vi "building_timbre.vi"() -> ()   [LabVIEW 2023]
uses:
  <vilib>/Analysis/3filter.llb/Filter Passband Type.ctl
  <vilib>/express/express analysis/Spectral/Block/exnSpectralBlock spectral measurements RMS poly.vi
  <vilib>/express/express analysis/Spectral/Block/exnSpectralBlock spectral measurements RMS WFM.vi
  <vilib>/express/express analysis/Spectral/XNode/ExpressSpectralMeasurementsBlockNode.xnode
  <vilib>/Analysis/NI_AALBase.lvlib
panel:
  out "Frequency Graph":cluster{"f0":dbl, "df":dbl, "magnitude":dbl[]}[](graph)
  in  "Duration (s)":dbl=1.0
  in  "Record Sound":bool
  in  "Open File":bool
  in  "path":path
  in  "Play Recorded Sound":bool
  in  "Play Sound":bool
  in  "stop":bool
  in  "Generated Signals":T1(array[cluster]) {"Signal" items=["Sine", "Square", "Triangle", "Sawtooth"]}
  in  "?":T3={"filter type"=enum."Lowpass", "low cutoff freq"=0.12500000000000006, "high cutoff freq"=0.45000000000000007} {"high cutoff freq" format="%0.2f"; "low cutoff freq" format="%0.4f"}
  in  "Filter OFF          Filter ON":bool
  out "Waveform Graph":waveform(dbl)[](graph)
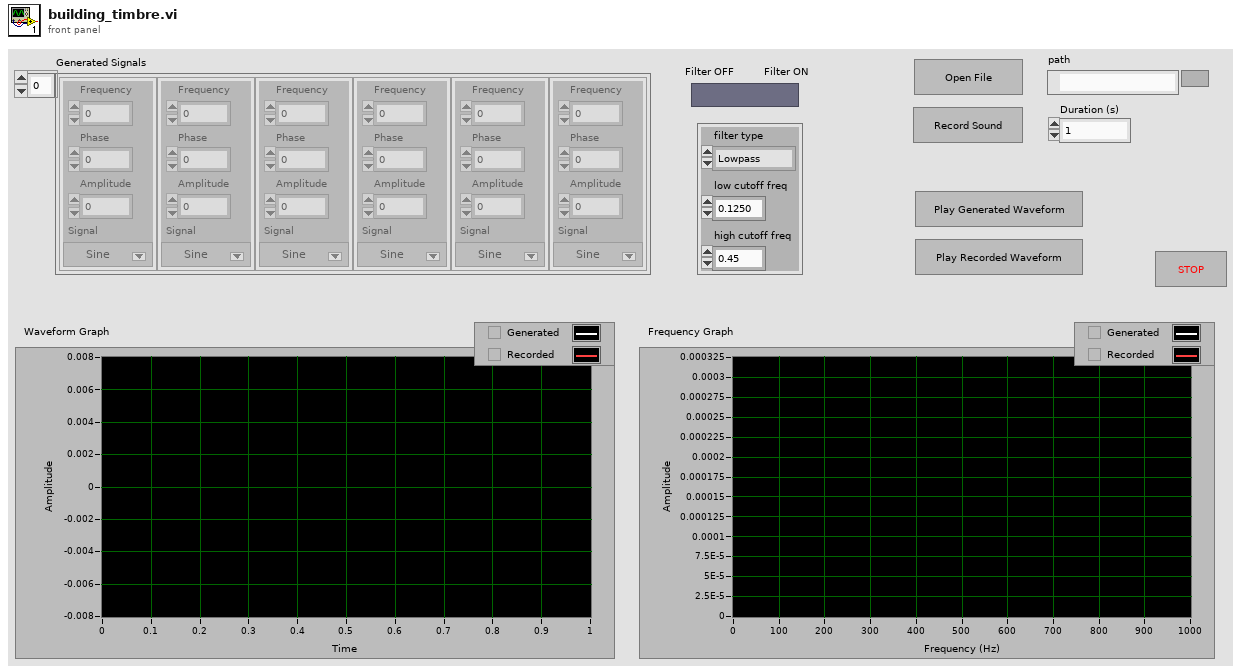
[diagram p1: front panel]
types:
  T1 = cluster{"Frequency":dbl, "Amplitude":dbl, "Signal":u16, "Phase":dbl}[]
  T2 = typedef "NI_AALBase.lvlib/Filter Passband Type.ctl" = enum32{"Lowpass", "Highpass", "Bandpass", "Bandstop"}
  T3 = cluster{"filter type":T2, "low cutoff freq":dbl, "high cutoff freq":dbl}
  T4 = cluster{"averaging mode":u16, "weighting mode":u16, "number of averages":u32}
  T5 = cluster{"dB On (F)":bool, "unwrap phase (F)":bool, "convert to degree (F)":bool}
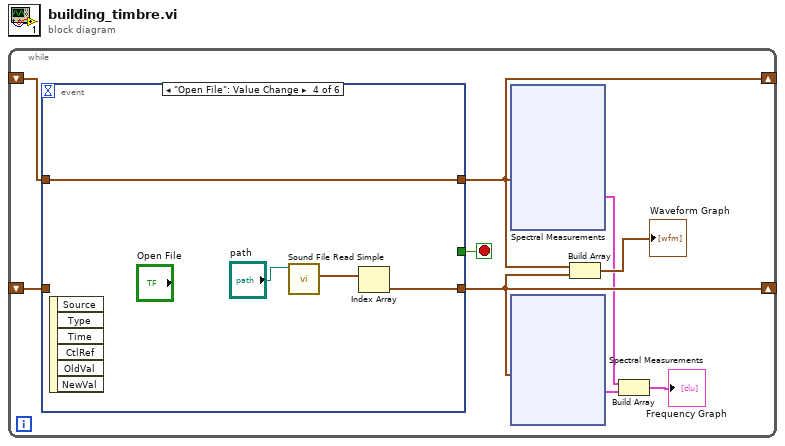
[diagram p0: block diagram]
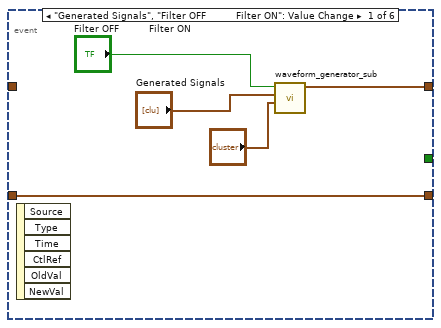
[diagram p2: hidden frame]
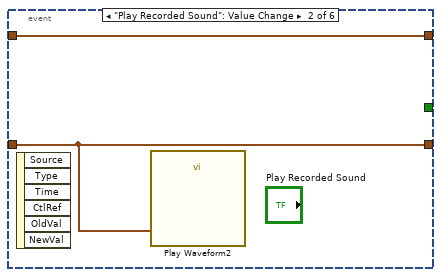
[diagram p3: hidden frame]
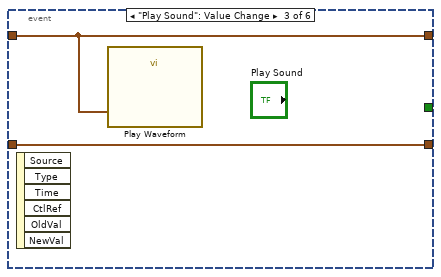
[diagram p4: hidden frame]
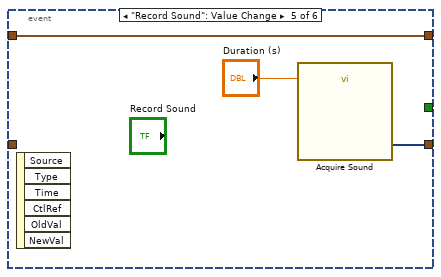
[diagram p5: hidden frame]
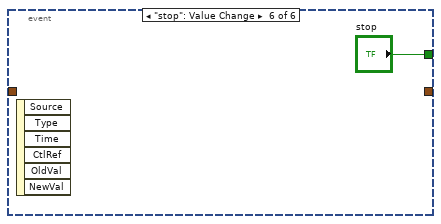
[diagram p6: hidden frame]
diagram:
  n1 = while {
    shift-right: [w6] -> _
    shift-left: _ -> [w8]
    shift-right: [w5] -> _
    shift-left: _ -> [w7]
    stop <- w9 stop-if-true
    n2 = event shown="[3] \"Open File\": Value Change" {
      selector: _ -> [_ _ _ _ _ _]
      dyn-events: _ -> [_ _ _ _ _ _]
      timeout: _ -> [_ _ _ _ _ _]
      tunnel: [w31 w36 w38 w39 w43 _] -> w6
      tunnel: [_ _ _ _ _ "stop"] -> w9
      tunnel: w8 -> [_ w36 w38 w39 w43 _]
      tunnel: [w30 w35 w37 w40 w44 _] -> w5
      tunnel: w7 -> [w30 w35 w37 _ _ _]
      event "Generated Signals", "Filter OFF          Filter ON": Value Change {
        n3 = event-data() -> ()  [unwired: 1 in, 6 out]
        n4 = call "waveform_generator_sub.vi"(9:"?", "Parameters"="Generated Signals", "Filter OFF   Filter ON"="Filter OFF          Filter ON") -> ("Waveform"=w31:waveform(dbl))  [unwired: 8 in]
      }
      event "Play Recorded Sound": Value Change {
        n5 = event-data() -> ()  [unwired: 1 in, 6 out]
        n6 = call "Play Waveform2"("Data"=w35) -> ()  [unwired: 18 in, 1 out]
      }
      event "Play Sound": Value Change {
        n7 = event-data() -> ()  [unwired: 1 in, 6 out]
        n8 = call "Play Waveform"("Data"=w38) -> ()  [unwired: 18 in, 1 out]
      }
      event "Open File": Value Change {
        n9 = event-data() -> ()  [unwired: 1 in, 6 out]
        n10 = call <vilib>:"Sound File Read Simple.vi"("path"="path") -> ("data"=w41:waveform(dbl)[])  [unwired: 7 in, 3 out]
        n11 = Index Array(array=w41) -> (element=w40:waveform(dbl))  [unwired: 1 in]
      }
      event "Record Sound": Value Change {
        n12 = event-data() -> ()  [unwired: 1 in, 6 out]
        n13 = call "Acquire Sound"("Duration (s)"="Duration (s)") -> ("Data"=w44:dynamicdata)  [unwired: 17 in, 1 out]
      }
      event "stop": Value Change {
        n14 = event-data() -> ()  [unwired: 1 in, 6 out]
      }
    }
    n15 = xnode "Spectral Measurements"("Signals"=w6) -> ("FFT - (RMS)"=w3:cluster{"f0":dbl, "df":dbl, "magnitude":dbl[]})  [unwired: 1 in, 2 out]
    n16 = xnode "Spectral Measurements"("Signals"=w5) -> ("FFT - (RMS)"=w2:cluster{"f0":dbl, "df":dbl, "magnitude":dbl[]})  [unwired: 1 in, 2 out]
    n17 = Build Array(w6, w5) -> (→"Waveform Graph":waveform(dbl)[])
    n18 = Build Array(w3, w2) -> (→"Frequency Graph":cluster{"f0":dbl, "df":dbl, "magnitude":dbl[]}[])
  }
